vi "SetValue.vi"(8 "error in (no error)":errorcluster, 10 "Value":string, 11 "DocumentClass in":refnum<class "Characteristic.lvclass">) -> (0 "error out":errorcluster, 3 "DocumentClass out":refnum<class "Characteristic.lvclass">)   [LabVIEW 2021, in "ProligentXMLGenerator.lvlib" / "Characteristic.lvclass"]
doc: "Set Value\n\nStore the value of the characteristic."
uses:
  Characteristic.lvclass
  Characteristic.lvclass/Characteristic.ctl
  Base/Attribute/Attribute.lvclass
  Base/String_2000/String_2000.lvclass
  C:/Projects/proligent-xml-generator-labview/src/ProligentXMLGenerator/Base/String/String.lvclass
  C:/Projects/proligent-xml-generator-labview/src/ProligentXMLGenerator/Base/Attribute/Attribute.lvclass
  C:/Projects/proligent-xml-generator-labview/src/ProligentXMLGenerator/Base/String_2000/String_2000.lvclass
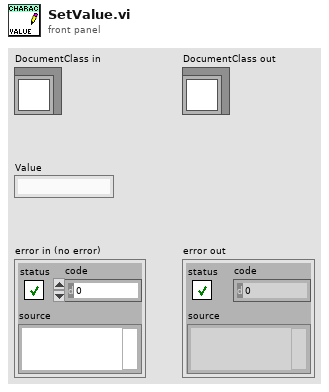
[diagram p1: front panel]
types:
  T1 = typedef "ProligentXMLGenerator.lvlib/Characteristic.lvclass/Data.ctl" = cluster{"Name":string, "CustomData":refnum<class "CustomData.lvclass">, "FullName":refnum<class "NonEmptyString_434.lvclass">, "Value":refnum<class "String_2000.lvclass">}
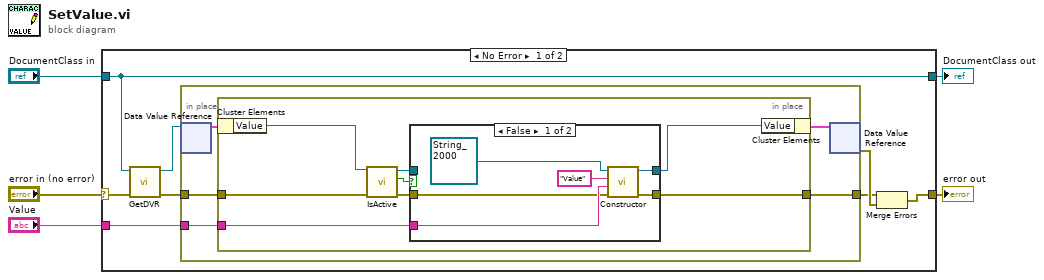
[diagram p0: block diagram]
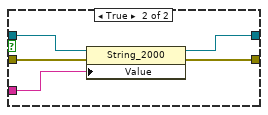
[diagram p2: hidden frame]
diagram:
  n1 = case shown="No Error" "error in (no error)" {
    selector: "error in (no error)" -> [w11 w38]
    tunnel: "DocumentClass in" -> [w6 w39]
    tunnel: [w8 w38] -> w4
    tunnel: "Value" -> [w7 _]
    tunnel: [w6 w39] -> w5
    frame No Error {
      n2 = call "GetDVR.vi"("error in"=w11, "Document in"=w6) -> ("error out"=w10:errorcluster, "DVRReference"=w12:refnum<data-value>)  [unwired: 8 in]
      n3 = in-place "In Place Element Structure" {
        in-place-border: w10 -> [w16]
        in-place-border: [w18] -> w9
        in-place-border: w7 -> [w17]
        n4 = in-place-dvr #1(w12) -> (w15:T1)  [unwired: 1 out]
        n5 = in-place "In Place Element Structure" {
          in-place-border: [w26] -> w18
          in-place-border: w17 -> [w25]
          in-place-border: w16 -> [w24]
          n6 = in-place-cluster #2(w15) -> ("Value"=w20:refnum<class "String_2000.lvclass">)
          n7 = call "IsActive.vi"("error in"=w24, "Attribute in"=w20) -> ("error out"=w21:errorcluster, "IsActive"=w22:bool, "Attribute in"=w23:refnum<class "String_2000.lvclass">)  [unwired: 7 in]
          n8 = case shown="False" w22 {
            tunnel: [w29 w37] -> w26
            tunnel: w25 -> [w31 w36]
            tunnel: w23 -> [_ w34]
            tunnel: w21 -> [w30 w35]
            tunnel: [w27 w33] -> w19
            frame False {
              n9 = call-dynamic "Constructor.vi"("error in"=w30, "Value"=w31, "Name"="Value", "String in"=refnum<class "String_2000.lvclass"> refnum ("IntegrationMetaData")) -> ("error out"=w29:errorcluster, "String out"=w27:refnum<class "String_2000.lvclass">)  [unwired: 6 in]
            }
            frame True {
              n10 = property on="Property Node" class="String_2000"(reference=w34, error in=w35, "Value"=w36) -> (reference out=w33:refnum<class "String_2000.lvclass">, error out=w37:errorcluster)
            }
          }
          n11 = in-place-cluster #2("Value"=w19) -> (w14:T1)
        }
        n12 = in-place-dvr #1(w14) -> (w13:errorcluster)  [unwired: 1 out]
      }
      n13 = Merge Errors(w9, w13) -> (w8:errorcluster)
    }
    frame Error {
    }
  }
  "error out" <- w4
  "DocumentClass out" <- w5
